vi "Read Status.vi"(8 "error in (no error)":errorcluster, 11 "Container in":refnum<class "Container.lvclass">) -> (0 "error out":errorcluster, 2 "Status":T1, 3 "Container out":refnum<class "Container.lvclass">)   [LabVIEW 2016, in "Container.lvclass"]
uses:
  Container.lvclass
  Container.lvclass/Container.ctl
  LFCSim/LFCSimShutt.lvclass
  ExtFlat/ExtFlatShutt.lvclass
  Sci/SciShutt.lvclass
  Solar/SolarShutt.lvclass
  SimFlat/SimFlatShutt.lvclass
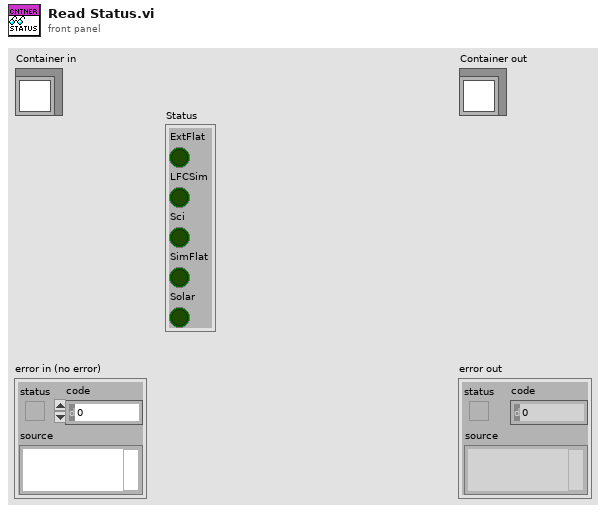
[diagram p1: front panel]
types:
  T1 = cluster{"ExtFlat":bool, "LFCSim":bool, "Sci":bool, "SimFlat":bool, "Solar":bool}
  T2 = cluster{"LFCSim":bool, "ExtFlat":bool, "Sci":bool, "Solar":bool, "SimFlat":bool}
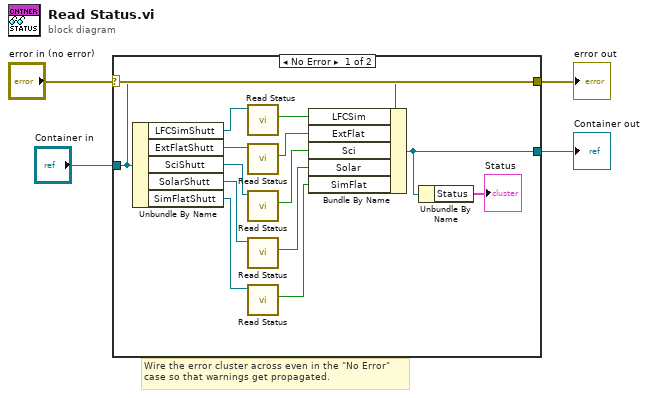
[diagram p0: block diagram]
diagram:
  # "Wire the error cluster across even in the \"No Error\"\ncase so that warnings get propagated."
  n1 = case shown="No Error" "error in (no error)" {
    selector: "error in (no error)" -> [w18 w20]
    tunnel: [w18 w20] -> w3
    tunnel: [w12 w19] -> w1
    tunnel: "Container in" -> [w10 w19]
    frame No Error {
      n2 = Unbundle By Name(w10) -> ("LFCSimShutt"=w8:refnum<class "LFCSimShutt.lvclass">, "ExtFlatShutt"=w9:refnum<class "ExtFlatShutt.lvclass">, "SciShutt"=w5:refnum<class "SciShutt.lvclass">, "SolarShutt"=w6:refnum<class "SolarShutt.lvclass">, "SimFlatShutt"=w7:refnum<class "SimFlatShutt.lvclass">)
      n3 = call-dynamic "Read Status.vi"("LFCSimShutt in"=w8) -> ("Status"=w16:bool)  [unwired: 8 in, 2 out]
      n4 = call-dynamic "Read Status.vi"("ExtFlatShutt in"=w9) -> ("Status"=w17:bool)  [unwired: 8 in, 2 out]
      n5 = call-dynamic "Read Status.vi"("SciShutt in"=w5) -> ("Status"=w15:bool)  [unwired: 8 in, 2 out]
      n6 = call-dynamic "Read Status.vi"("SolarShutt in"=w6) -> ("Status"=w14:bool)  [unwired: 8 in, 2 out]
      n7 = call-dynamic "Read Status.vi"("SimFlatShutt in"=w7) -> ("Status"=w13:bool)  [unwired: 8 in, 2 out]
      n8 = Bundle By Name(cluster=w10, "LFCSim"=w16, "ExtFlat"=w17, "Sci"=w15, "Solar"=w14, "SimFlat"=w13) -> (w12:refnum<class "Container.lvclass">)
      n9 = Unbundle By Name(w12) -> ("Status"=→"Status":T2)
    }
    frame Error {
    }
  }
  "error out" <- w3
  "Container out" <- w1
